vi "is valid websocket header.vi"(10 "parameters":T2, 11 "headers":T1) -> (1 "supported protocols":string[](array[string]), 2 "return sec key":string, 3 "valid websocket headers":bool, 5 "host field":string)   [LabVIEW 2016, in "websocket standalone server.lvclass"]
uses:
  websocket standalone server.lvclass
  websocket connection parameters.ctl
  HTTP headers/http header data.ctl
  HTTP headers/http headers.lvlib
  websocket core.lvlib
panel:
  out "origin":string
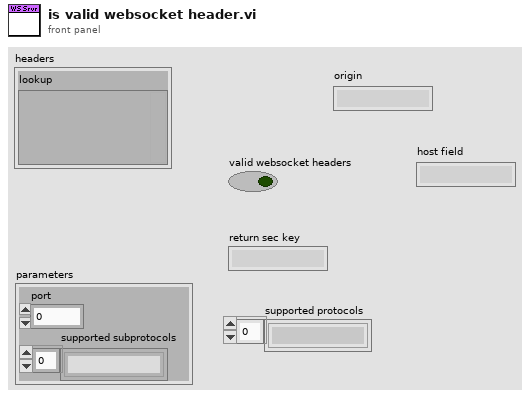
[diagram p1: front panel]
types:
  T1 = typedef "http headers.lvlib/http header data.ctl" = cluster{"lookup":variant}
  T2 = typedef "websocket standalone server.lvclass/websocket connection parameters.ctl" = cluster{"port":u16, "supported subprotocols":string[]}
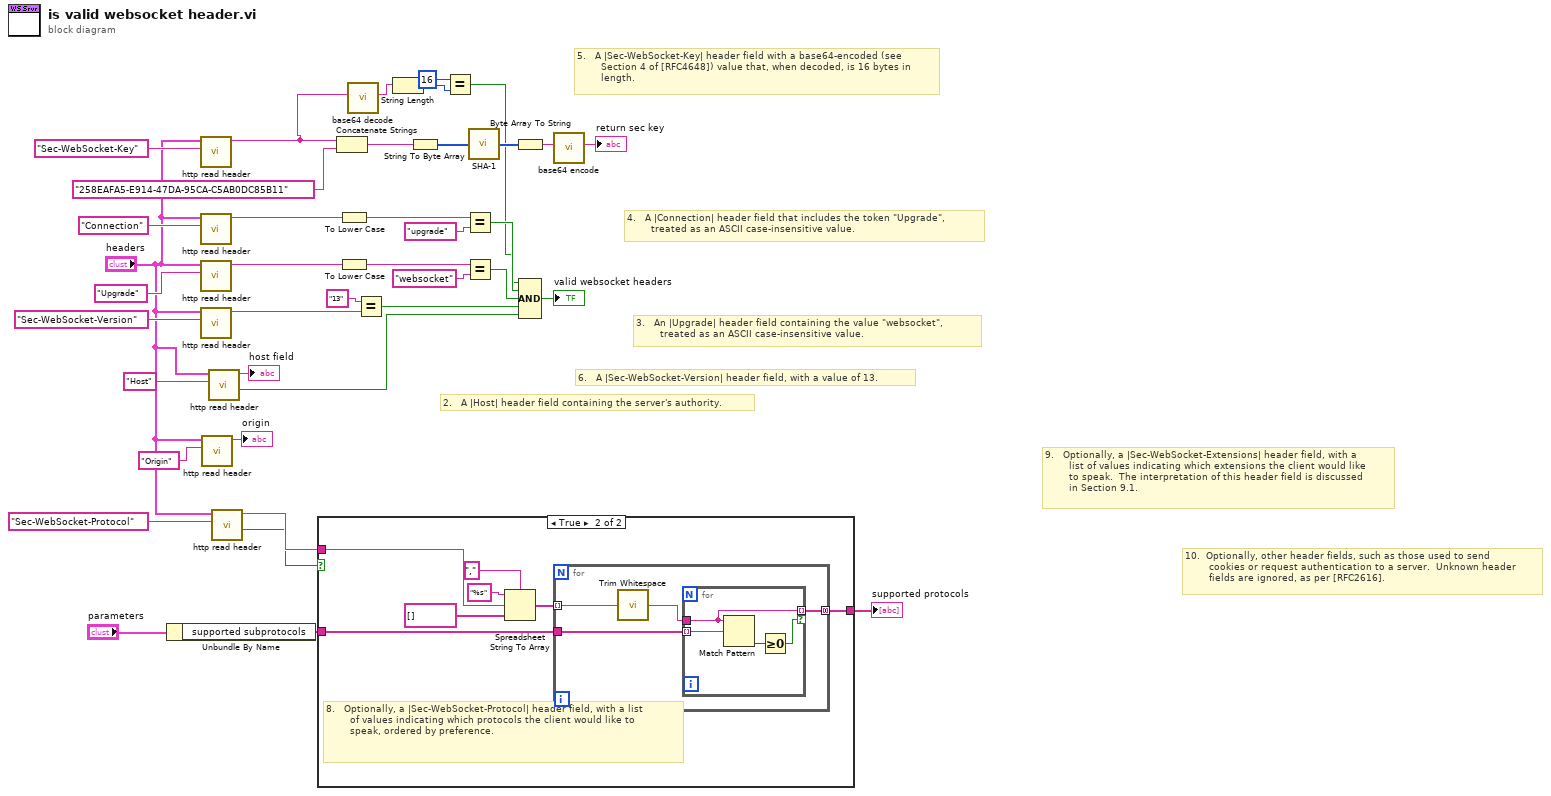
[diagram p0: block diagram]
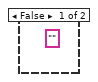
[diagram p2: hidden frame]
diagram:
  # "10.  Optionally, other header fields, such as those used to send\n        cookies or request authentication to a server.  Unknown header\n        fields are ignored, as per [RFC2616]."
  # "9.   Optionally, a |Sec-WebSocket-Extensions| header field, with a\n        list of values indicating which extensions the client would like\n        to speak.  The interpretation of this header field is discussed\n        in Section 9.1."
  # "6.   A |Sec-WebSocket-Version| header field, with a value of 13."
  # "2.   A |Host| header field containing the server's authority."
  # "3.   An |Upgrade| header field containing the value \"websocket\",\n        treated as an ASCII case-insensitive value."
  # "4.   A |Connection| header field that includes the token \"Upgrade\",\n        treated as an ASCII case-insensitive value."
  # "5.   A |Sec-WebSocket-Key| header field with a base64-encoded (see\n        Section 4 of [RFC4648]) value that, when decoded, is 16 bytes in\n        length."
  n1 = Unbundle By Name("parameters") -> ("supported subprotocols"=w37:string[])
  n2 = call "http read header.vi"("header field name"="Sec-WebSocket-Key", "headers"="headers") -> ("value"=w8:string)  [unwired: 8 in, 1 out]
  n3 = call "http read header.vi"("header field name"="Connection", "headers"="headers") -> ("value"=w18:string)  [unwired: 8 in, 1 out]
  n4 = call "http read header.vi"("header field name"="Upgrade", "headers"="headers") -> ("value"=w23:string)  [unwired: 8 in, 1 out]
  n5 = call "http read header.vi"("header field name"="Sec-WebSocket-Version", "headers"="headers") -> ("value"=w29:string)  [unwired: 8 in, 1 out]
  n6 = call "http read header.vi"("header field name"="Origin", "headers"="headers") -> ("value"=→"origin":string)  [unwired: 8 in, 1 out]
  n7 = call "http read header.vi"("header field name"="Host", "headers"="headers") -> ("found"=w10:bool, "value"=→"host field":string)  [unwired: 8 in]
  n8 = call "http read header.vi"("header field name"="Sec-WebSocket-Protocol", "headers"="headers") -> ("found"=w35:bool, "value"=w36:string)  [unwired: 8 in]
  n9 = case shown="True" w35 {
    tunnel: w36 -> [_ w45]
    tunnel: w37 -> [_ w43]
    tunnel: [_ w40] -> w12
    frame False {
      (unwired) "" ("trimmed string")
    }
    frame True {
      # "8.   Optionally, a |Sec-WebSocket-Protocol| header field, with a list\n        of values indicating which protocols the client would like to\n        speak, ordered by preference."
      n10 = Spreadsheet String To Array(delimiter (Tab)=",", format string="%s", spreadsheet string=w45, array type (2D Dbl)=string[] []) -> (array=w44:string[])
      n11 = for {
        tunnel: w44 -> [w49] mode=indexing
        tunnel: [w47] -> w40 mode=concatenating
        tunnel: w43 -> [w50]
        n12 = call <vilib>:"Trim Whitespace.vi"("string"=w49) -> ("trimmed string"=w48:string)  [unwired: 1 in]
        n13 = for {
          tunnel: w50 -> [w54] mode=indexing
          tunnel: w48 -> [w53]
          tunnel: [w53] -> w47 mode=indexing if=w51
          n14 = Match Pattern(string=w53, regular expression=w54) -> (offset past match=w52:i32)  [unwired: 1 in, 3 out]
          n15 = Greater Or Equal To 0?(x=w52) -> (x >= 0?=w51:bool)
        }
      }
    }
  }
  "supported protocols" <- w12
  n16 = Concatenate Strings(w8, "258EAFA5-E914-47DA-95CA-C5AB0DC85B11") -> (w25:string)
  n17 = To Lower Case(string=w18) -> (all lower case string=w19:string)
  n18 = To Lower Case(string=w23) -> (all lower case string=w22:string)
  n19 = call "base64 decode.vi"("string in (base64-encoded)"=w8) -> ("string out (decoded)"=w7:string)  [unwired: 9 in, 1 out]
  n20 = Equal?(x="13" ("y"), y=w29) -> (x = y?=w33:bool)
  n21 = String Length(string=w7) -> (length=w6:i32)
  n22 = String To Byte Array(string=w25) -> (unsigned byte array=w26:u8[])
  n23 = Equal?(x=16, y=w6) -> (x = y?=w4:bool)
  n24 = Equal?(x=w19, y="upgrade") -> (x = y?=w31:bool)
  n25 = Equal?(x=w22, y="websocket") -> (x = y?=w32:bool)
  n26 = call "SHA-1.vi"("Data"=w26) -> ("message-digest"=w27:u8[])
  n27 = Byte Array To String(unsigned byte array=w27) -> (string=w28:string)
  n28 = Compound Arithmetic op=AND(w4, w31, w32, w33, w10) -> (→"valid websocket headers":bool)
  n29 = call "base64 encode.vi"("string in (not encoded)"=w28) -> ("string out (base64-encoded)"=→"return sec key":string)  [unwired: 10 in]
